vi "Write Ip addr.vi"(8 "error in (no error)":errorcluster, 10 "IP address":T1, 11 "MB Param in":refnum<class "TCP Param.lvclass">) -> (0 "error out":errorcluster, 3 "MB Param out":refnum<class "TCP Param.lvclass">)   [LabVIEW 2021, in "Param.lvlib" / "TCP Param.lvclass"]
uses:
  TCP Param.lvclass
  TCP Param.lvclass/TCP Param.ctl
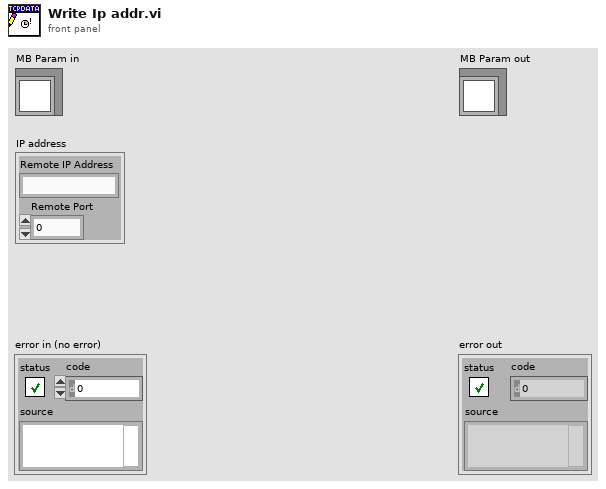
[diagram p1: front panel]
types:
  T1 = cluster{"Remote IP Address":string, "Remote Port":u16}
  T2 = typedef "Param.lvlib/TCP Param.lvclass/timeouts.ctl" = cluster{"conn_timeout":i32, "reconn_timeout":i32, "N attempt max":i32, "t_reset_TTL":i32, "write_timeout":i32, "read_timeout":i32, "period":i32}
  T3 = cluster{"IP address":cluster{"Remote IP Address":string, "Remote Port":u16}, "timeouts":T2}
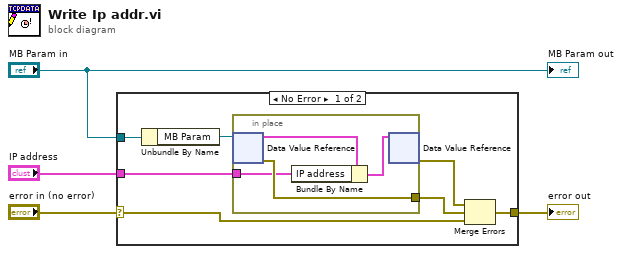
[diagram p0: block diagram]
diagram:
  n1 = case shown="No Error" "error in (no error)" {
    selector: "error in (no error)" -> [w6 w16]
    tunnel: [w10 w16] -> w3
    tunnel: "MB Param in" -> [w11 _]
    tunnel: "IP address" -> [w5 _]
    frame No Error {
      n2 = Unbundle By Name(w11) -> ("MB Param"=w7:refnum<data-value>)
      n3 = in-place {
        in-place-border: [w15] -> w8
        in-place-border: w5 -> [w12]
        n4 = in-place-dvr #1(w7) -> (w14:T3, w15:errorcluster)
        n5 = Bundle By Name(cluster=w14, "IP address"=w12) -> (w13:T3)
        n6 = in-place-dvr #1(w13) -> (w9:errorcluster)  [unwired: 1 out]
      }
      n7 = Merge Errors(w9, w8, w6) -> (w10:errorcluster)
    }
    frame Error {
    }
  }
  "error out" <- w3
  "MB Param out" <- "MB Param in"
